vi "GetVIName.vi"(6 "error in":errorcluster, 9 "VI Interpreter in":refnum<class "VI Interpreter.lvclass">) -> (0 "error out":errorcluster, 3 "VI Interpreter out":refnum<class "VI Interpreter.lvclass">, 4 "VI Name":string)   [LabVIEW 2014, in "VI Interpreter.lvclass"]
uses:
  VI Interpreter.lvclass
  VI Interpreter.lvclass/VI Interpreter.ctl
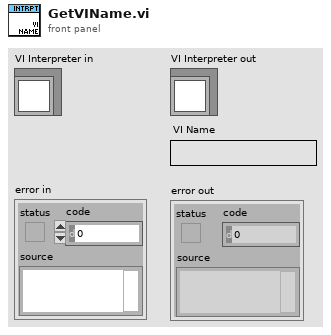
[diagram p1: front panel]
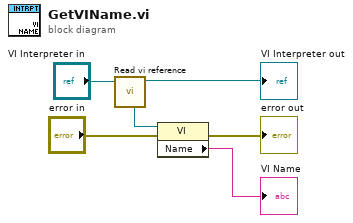
[diagram p0: block diagram]
diagram:
  n1 = call "Read vi reference.vi"("VI Interpreter in"="VI Interpreter in") -> ("VI Interpreter out"=→"VI Interpreter out":refnum<class "VI Interpreter.lvclass">, "vi reference"=w5:refnum<vi>)  [unwired: 7 in]
  n2 = property class="VI"(reference=w5, error in="error in") -> (error out=→"error out":errorcluster, "Name"=→"VI Name":string)  [unwired: 1 out]
